vi "LVFunction_Imop_WavefrontCorrectorSetupFile_GetInformation.vi"(0 "module path":path, 11 "error in (no error)":errorcluster) -> (6 "ConfigMiroir":T1={"Mirror name"="", "Plugin name"="", "Serial number"="", "Revision"="", "Number of commands"=0, "Sleep after command apply (ms)"=0, "Has internal memory ?"=TRUE}, 15 "error out":errorcluster)   [LabVIEW 2020]
uses:
  WavefrontCorrectorSpecifications.ctl
  WavefrontCorrectorSet.lvclass
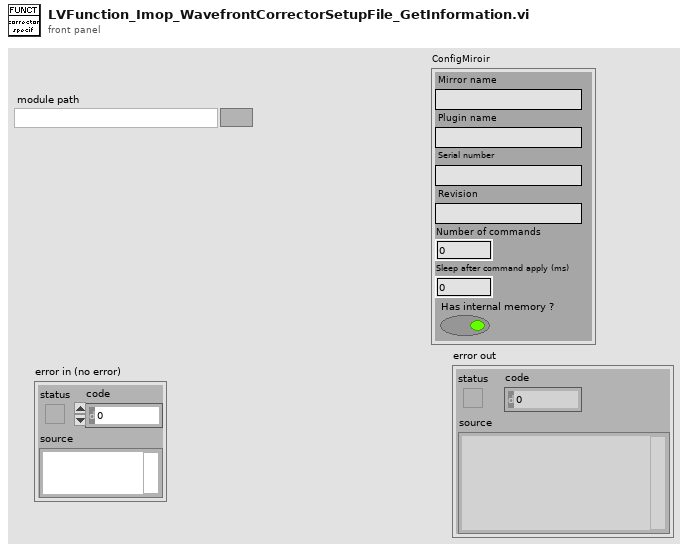
[diagram p1: front panel]
types:
  T1 = typedef "WavefrontCorrectorSpecifications.ctl" = cluster{"Mirror name":string, "Plugin name":string, "Serial number":string, "Revision":string, "Number of commands":i32, "Sleep after command apply (ms)":i32, "Has internal memory ?":bool}
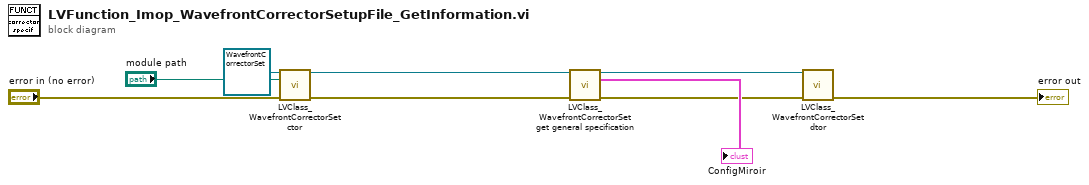
[diagram p0: block diagram]
diagram:
  n1 = call "LVClass_WavefrontCorrectorSet ctor.vi"("WavefrontCorrectorSet in"=refnum<class "WavefrontCorrectorSet.lvclass"> refnum, "PathToWavefrontCorrectorSetupFile"="module path", "error in (no error)"="error in (no error)") -> ("WavefrontCorrectorSet out"=w6:refnum<class "WavefrontCorrectorSet.lvclass">, "error out"=w4:errorcluster)  [unwired: 11 in]
  n2 = call "LVClass_WavefrontCorrectorSet get general specification.vi"("WavefrontCorrectorSet in"=w6, "error in (no error)"=w4) -> ("WavefrontCorrectorSet out"=w5:refnum<class "WavefrontCorrectorSet.lvclass">, "ConfigMiroir"=→"ConfigMiroir":T1, "error out"=w2:errorcluster)  [unwired: 11 in]
  n3 = call "LVClass_WavefrontCorrectorSet dtor.vi"("WavefrontCorrectorSet in"=w5, "error in (no error)"=w2) -> ("error out"=→"error out":errorcluster)  [unwired: 12 in, 1 out]
